vi "TiePie.Scp.ScpConnectionTest.vi"() -> ()   [LabVIEW 2013, in "LVTiePie.lvlib"]
uses:
  LVTiePie.lvlib
  PAN/LabVEW/Tie Pie/bin/libtiepie.dll
  TiePie.Gen.handle.ctl
panel:
  out "return type":u8
  out "GenHandle out":T1
  in  "GenHandle":T1
  out "error out":errorcluster
  in  "error in (no error)":errorcluster
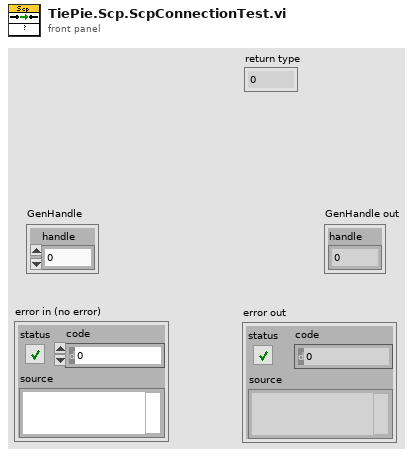
[diagram p1: front panel]
types:
  T1 = typedef "TiePie.Gen.handle.ctl" = cluster{"handle":u32}
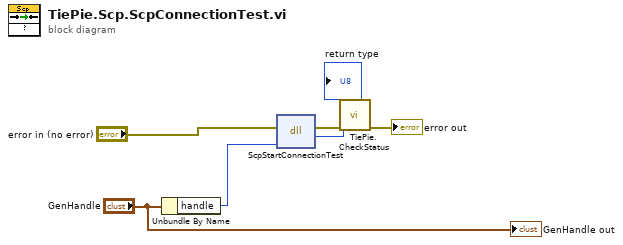
[diagram p0: block diagram]
diagram:
  n1 = Unbundle By Name("GenHandle") -> ("handle"=w5:u32)
  n2 = dll-call lib="C:/Users/mbirski/Desktop/PAN/LabVEW/Tie Pie/bin/libtiepie.dll" fn="ScpStartConnectionTest"(error in="error in (no error)", "handle"=w5) -> (error out=w3:errorcluster, "isConnectionTestStarted"=→"return type":u8)  [unwired: 3 in, 1 out]
  n3 = call "TiePie.CheckStatus.vi"("error in (no error)"=w3) -> ("error out"=→"error out":errorcluster)  [unwired: 10 in]
  "GenHandle out" <- "GenHandle"
